vi "move2mark (SubVI).vi"(9 "index":i32, 11 "Application in":refnum<vi>) -> (3 "Application out":refnum<vi>)   [LabVIEW 2021]
uses:
  <userlib>/Nanonis Prog Interface V5/Nanonis Prog Interface.lvlib
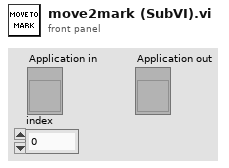
[diagram p1: front panel]
types:
  T1 = cluster{"X (m)":sgl, "Y (m)":sgl, "Text":string, "Color":u32, "Visible":bool}[]
  T2 = cluster{"X (m)":sgl, "Y (m)":sgl, "Text":string, "Color":u32, "Visible":bool}
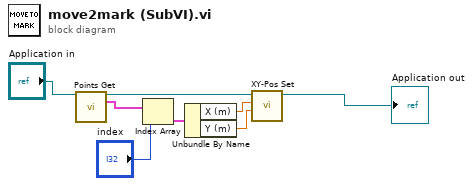
[diagram p0: block diagram]
diagram:
  n1 = call <userlib>:"Points Get.vi"("Application ref in"="Application in") -> ("Application ref out"=w5:refnum<vi>, "Points"=w3:T1)  [unwired: 12 in, 1 out]
  n2 = Index Array(array=w3, index="index") -> (element=w4:T2)
  n3 = Unbundle By Name(w4) -> ("X (m)"=w6:sgl, "Y (m)"=w7:sgl)
  n4 = call <userlib>:"XY-Pos Set.vi"("Y (m)"=w7, "X (m)"=w6, "Application ref in"=w5) -> ("Application ref out"=→"Application out":refnum<vi>)  [unwired: 5 in, 1 out]
